vi "Write C.vi"(8 "error in (no error)":errorcluster, 10 "C":dbl, 11 "Arithmetic in":refnum<class "Arithmetic.lvclass">) -> (0 "error out":errorcluster, 3 "Arithmetic out":refnum<class "Arithmetic.lvclass">)   [LabVIEW 2023, in "Arithmetic.lvclass"]
uses:
  Arithmetic.lvclass
  Arithmetic.lvclass/Arithmetic.ctl
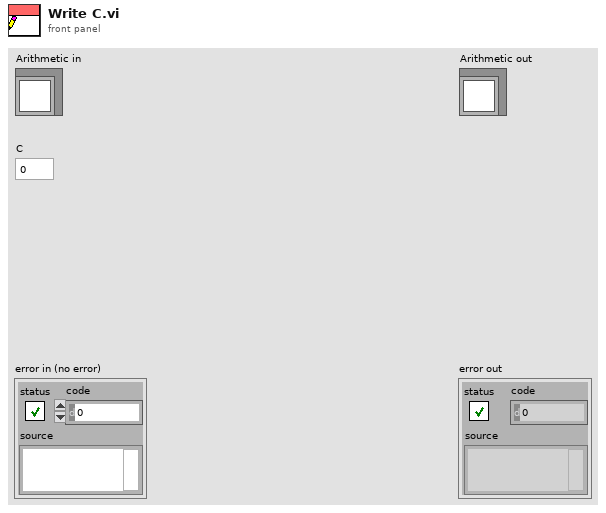
[diagram p1: front panel]
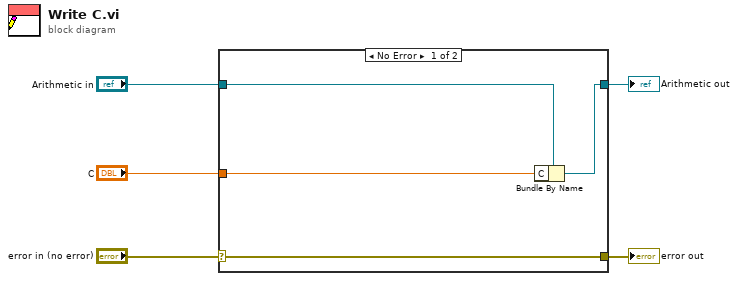
[diagram p0: block diagram]
diagram:
  n1 = case shown="No Error" "error in (no error)" {
    selector: "error in (no error)" -> [w9 w10]
    tunnel: [w9 w10] -> w4
    tunnel: [w7 w11] -> w2
    tunnel: "Arithmetic in" -> [w8 w11]
    tunnel: "C" -> [w6 _]
    frame No Error {
      n2 = Bundle By Name(cluster=w8, "C"=w6) -> (w7:refnum<class "Arithmetic.lvclass">)
    }
    frame Error {
    }
  }
  "error out" <- w4
  "Arithmetic out" <- w2
